vi "AMX-CCDA获取图像.vi"(7 "Session Out CCD2":T1, 8 "error in (no error)":errorcluster caption="错误输入（无错误）", 10 "Image Name":string="I1", 11 "ParamsUI":T2={"IsNorImage"=FALSE, "Exposure Values"=500, "ImagePath"=path "C:/Users/hedongpo/Desktop/514-hdp/Alignment Assemble System/Test Picture/B/3.bmp"} caption="参数界面" {"Exposure Values" scale=0.0..200000.0}) -> (0 "error out":errorcluster={"status"=TRUE, "code"=-1074360316, "source"="AMX-CCD1获取图像.vi->LabVIEW Function Structure.vi中的属性节点 (arg 1)"} caption="错误输出", 2 "Session Out":T1, 3 "Image out":T3(plugin-control), 4 "数值":dbl)   [LabVIEW 2017]
uses:
  <vilib>/userdefined/High Color/IMAQdx.ctl
  <vilib>/vision/driver/IMAQdx.llb/IMAQdx Buffer Number Mode.ctl
  Global System.vi
  <resource>/objmgr/imaqdx.rc
  <vilib>/vision/driver/NI_Vision_Acquisition_Software.lvlib
  <vilib>/vision/NI_Vision_Development_Module.lvlib
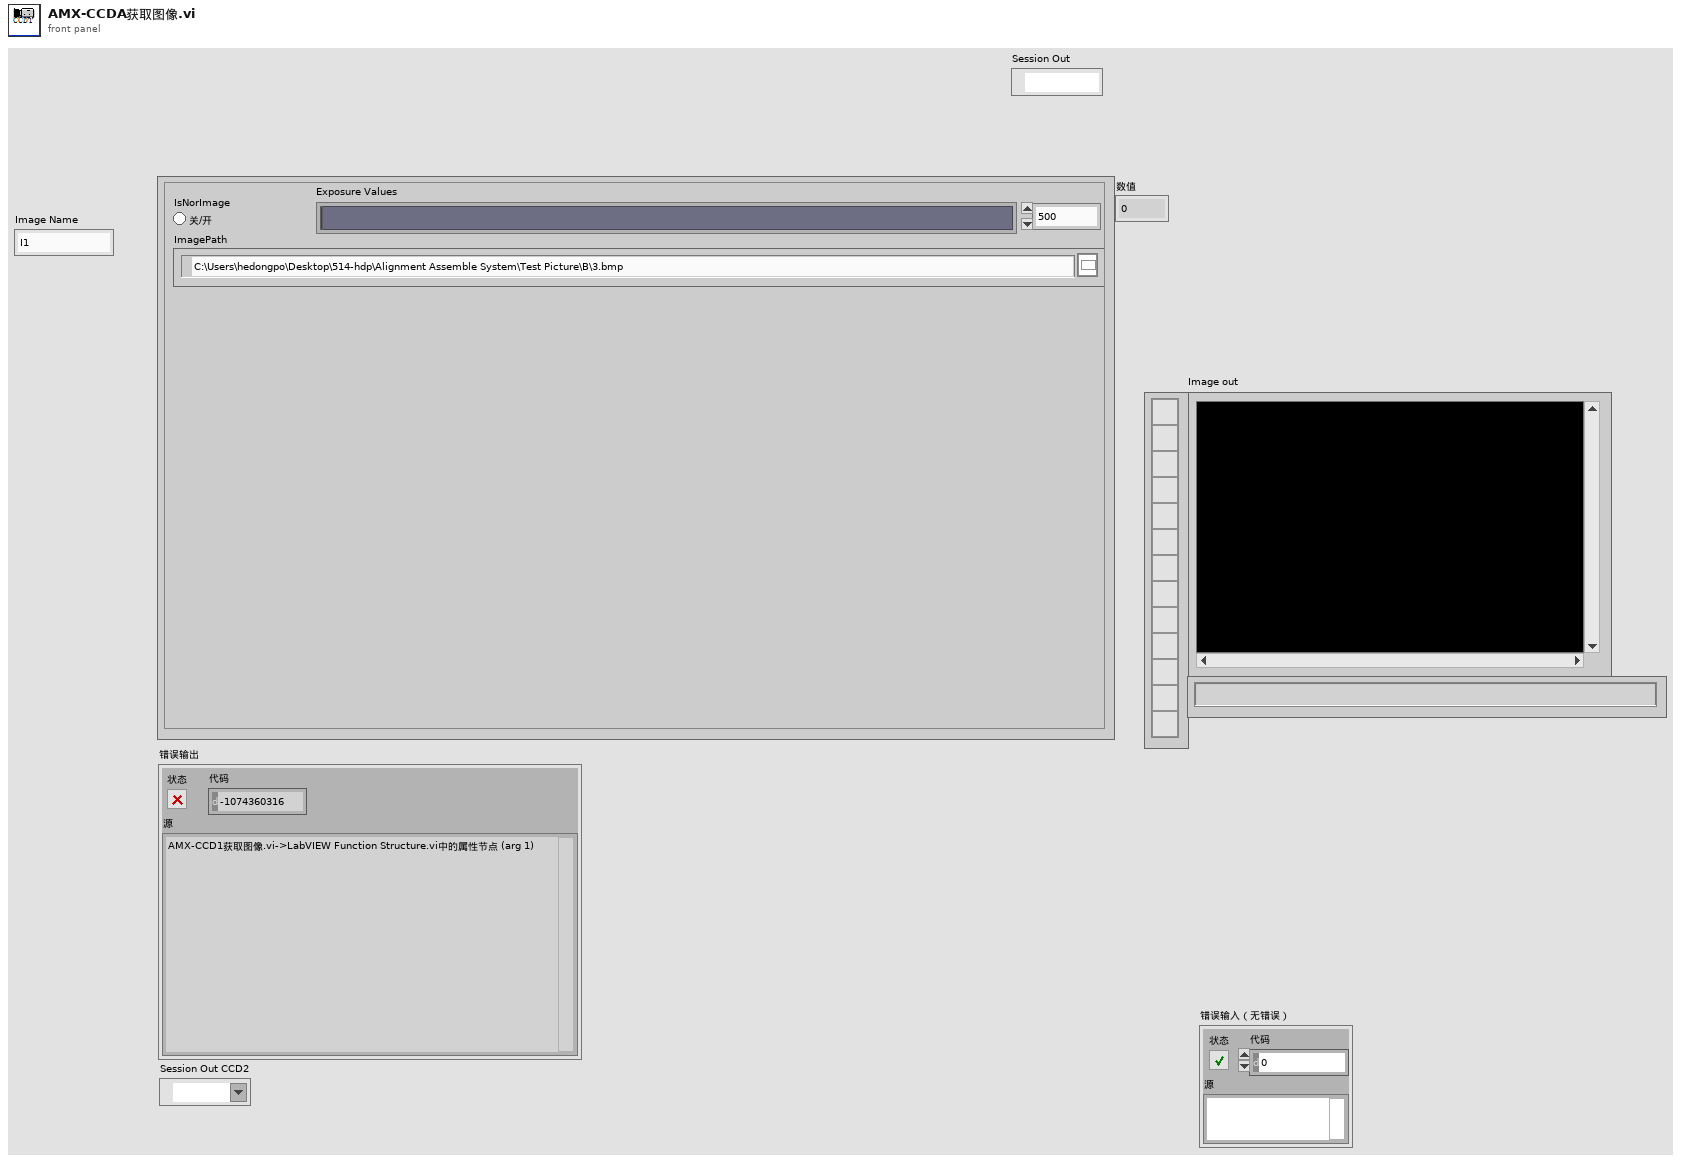
[diagram p1: front panel]
types:
  T1 = typedef "IMAQdx.ctl" = refnum<k21>
  T2 = cluster{"IsNorImage":bool, "Exposure Values":i64, "ImagePath":path}
  T3 = typedef "IMAQ Image.ctl" = refnum<image>
  T4 = typedef "Image Type" = u32
  T5 = typedef "NI_Vision_Acquisition_Software.lvlib/IMAQdx Buffer Number Mode.ctl" = enum32{"Next", "Last", "Buffer Number", "Every", "Last New"}
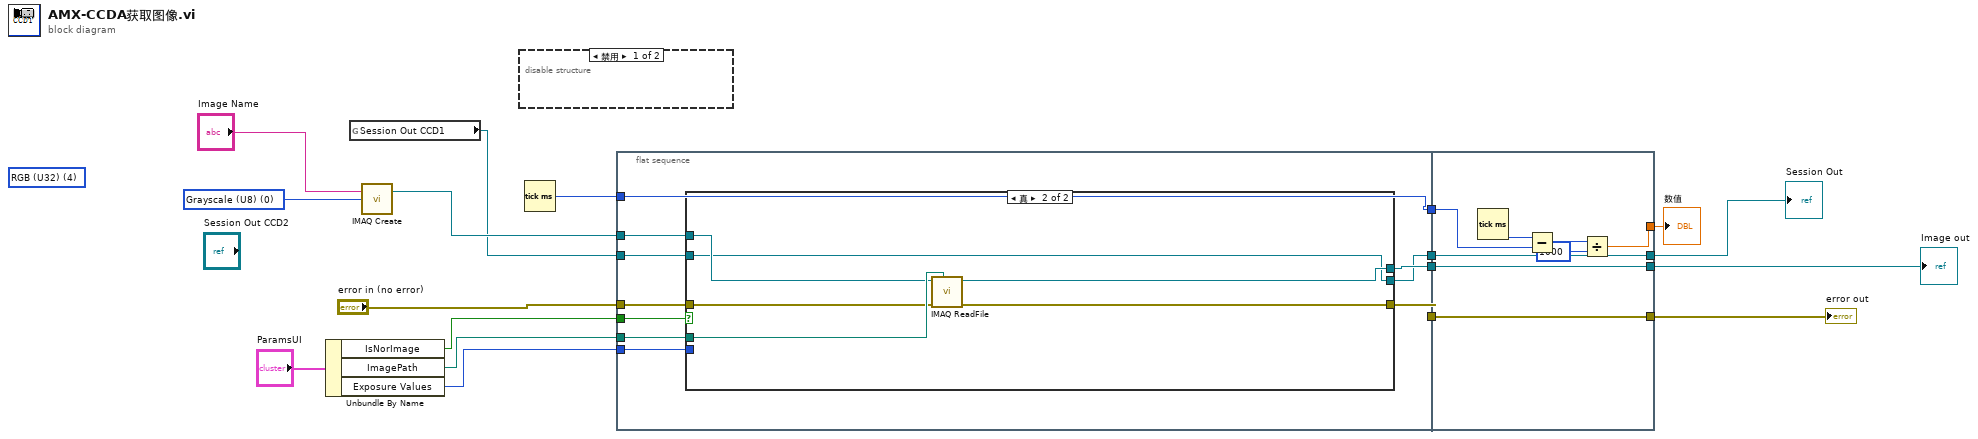
[diagram p0: block diagram]
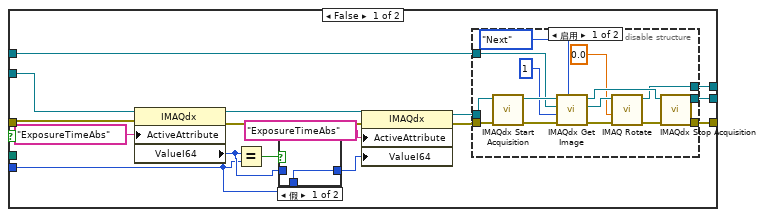
[diagram p3: hidden frame]
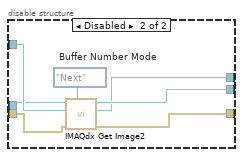
[diagram p5: hidden frame]
diagram:
  (unwired) T4 4 items=["Grayscale (U8)", "Grayscale (I16)", "Grayscale (SGL)", "Complex (CSG)", "RGB (U32)", "HSL (U32)", "RGB (U64)", "Grayscale (U16)"] ("Image Type")
  w13 = T4 0 items=["Grayscale (U8)", "Grayscale (I16)", "Grayscale (SGL)", "Complex (CSG)", "RGB (U32)", "HSL (U32)", "RGB (U64)", "Grayscale (U16)"] ("Image Type")
  n1 = Unbundle By Name("ParamsUI") -> ("IsNorImage"=w3:bool, "ImagePath"=w2:path, "Exposure Values"=w18:i64)
  n2 = global read "Global System.vi" "Session Out CCD1"() -> (w1:T1)
  n3 = call "IMAQ Create"("Image Name"="Image Name", "Image Type"=w13) -> ("New Image"=w16:T3)  [unwired: 3 in, 1 out]
  n4 = disable-structure shown="禁用" {
    frame Disabled {
    }
    frame Enabled {
    }
  }
  n5 = Tick Count (ms)() -> (millisecond timer value=w9:u32)
  n6 = flat-sequence {
    tunnel: w3 -> [w28]
    tunnel: w2 -> [w27]
    tunnel: w18 -> [w26]
    tunnel: w16 -> [w25]
    tunnel: "error in (no error)" -> [w24]
    tunnel: w1 -> [w21]
    tunnel: w9 -> [w19]
    tunnel: [w23] -> w8
    tunnel: [w22] -> w7
    tunnel: [w20] -> w6
    tunnel: [w19] -> w5
    tunnel: [w80] -> w10
    tunnel: [w81] -> w11
    tunnel: [w82] -> w14
    tunnel: w8 -> [w82]
    tunnel: w7 -> [w81]
    tunnel: w6 -> [w80]
    tunnel: w5 -> [w78]
    tunnel: [w75] -> w4
    frame #0 {
      n7 = case shown="真" w28 {
        tunnel: w27 -> [_ w74]
        tunnel: [w43 w73] -> w22
        tunnel: w26 -> [w29 _]
        tunnel: w21 -> [w37 w69]
        tunnel: w25 -> [w44 w72]
        tunnel: w24 -> [w34 w71]
        tunnel: [w41 w70] -> w23
        tunnel: [w42 w69] -> w20
        frame False {
          n8 = property class="IMAQdx"(reference=w37, error in=w34, "ActiveAttribute"="ExposureTimeAbs") -> (reference out=w36:T1, error out=w35:errorcluster, "ValueI64"=w30:i64)
          n9 = Equal?(x=w30, y=w29) -> (x = y?=w32:bool)
          n10 = case shown="假" w32 {
            tunnel: [w45 w46] -> w31
            tunnel: w30 -> [_ w46]
            tunnel: w29 -> [w45 _]
            frame False {
            }
            frame True {
            }
          }
          n11 = property class="IMAQdx"(reference=w36, error in=w35, "ActiveAttribute"="ExposureTimeAbs", "ValueI64"=w31) -> (reference out=w40:T1, error out=w39:errorcluster)
          n12 = disable-structure shown="启用" {
            disable-tunnel: w44 -> [w52 w67]
            disable-tunnel: [w51 w63] -> w43
            disable-tunnel: [w50 w64] -> w42
            disable-tunnel: [w49 w62] -> w41
            disable-tunnel: w40 -> [w48 w66]
            disable-tunnel: w39 -> [w47 w65]
            frame Enabled {
              n13 = call <vilib>:"IMAQdx Start Acquisition.vi"("error in"=w47, "Session In"=w48) -> ("error out"=w60:errorcluster, "Session Out"=w61:T1)  [unwired: 8 in]
              n14 = call <vilib>:"IMAQdx Get Image.vi"("Buffer Number Mode (Next)"=IMAQdx_Buffer_Number_Mode."Next", "error in"=w60, "Buffer Number In"=u32 1, "Image In"=w52, "Session In"=w61) -> ("error out"=w55:errorcluster, "Image Out"=w56:T3, "Session Out"=w57:T1)  [unwired: 3 in, 1 out]
              n15 = call "IMAQ Rotate"("error in (no error)"=w55, "Angle (degrees)"=sgl 0.0, "Image Src"=w56) -> ("error out"=w54:errorcluster, "Image Dst Out"=w51:T3)  [unwired: 7 in]
              n16 = call <vilib>:"IMAQdx Stop Acquisition.vi"("error in"=w54, "Session In"=w57) -> ("error out"=w49:errorcluster, "Session Out"=w50:T1)  [unwired: 8 in]
            }
            frame Disabled {
              w68 = IMAQdx_Buffer_Number_Mode."Next"  # Buffer Number Mode
              n17 = call <vilib>:"IMAQdx Get Image2.vi"("Buffer Number Mode (Next)"=w68, "error in"=w65, "Image In"=w67, "Session In"=w66) -> ("error out"=w62:errorcluster, "Image Out"=w63:T3, "Session Out"=w64:T1)  [unwired: 4 in, 1 out]
            }
          }
        }
        frame True {
          n18 = call "IMAQ ReadFile"("File Path"=w74, "error in (no error)"=w71, "Image"=w72) -> ("error out"=w70:errorcluster, "Image Out"=w73:T3)  [unwired: 4 in, 3 out]
        }
      }
    }
    frame #1 {
      n19 = Tick Count (ms)() -> (millisecond timer value=w79:u32)
      n20 = Subtract(x=w79, y=w78) -> (x-y=w77:u32)
      n21 = Divide(x=w77, y=u32 1000) -> (x/y=w75:dbl)
    }
  }
  "Image out" <- w11
  "error out" <- w14
  "Session Out" <- w10
  "数值" <- w4
